vi "Auto Loop 4.vi"(2 "Auto State":u8, 3 "Call Context":T1) -> (1 "SubState 5":T2)   [LabVIEW 2014]
uses:
  typedefs/state machine/singleUseSubstate.ctl
  <vilib>/Rock Robotics/WPI/DriverStation/WPI_DriverStationDerivedRobotMode.ctl
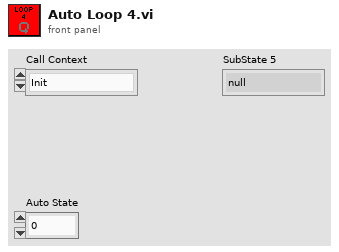
[diagram p1: front panel]
types:
  T1 = typedef "WPI_DriverStationDerivedRobotMode.ctl" = enum16{"Init", "Execute", "Stop"}
  T2 = typedef "singleUseSubstate.ctl" = enum16{"null", "wait", "shift high", "shift low", "end"}
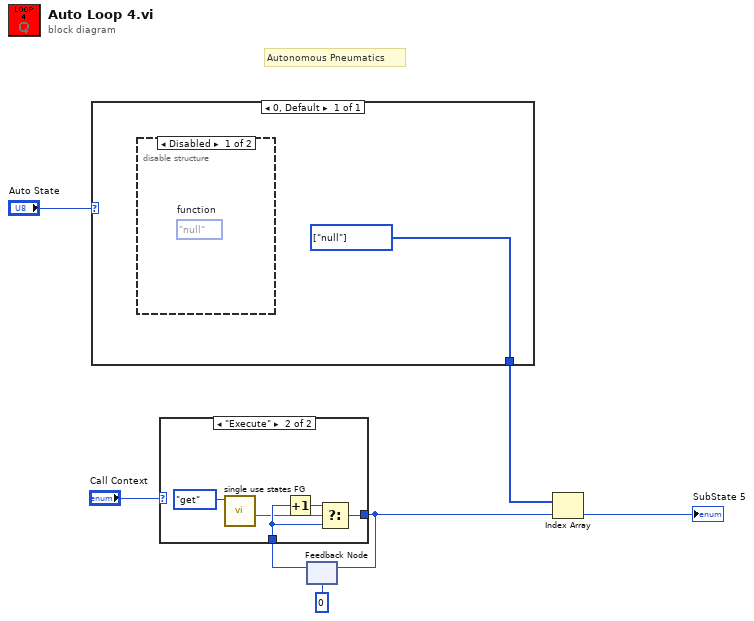
[diagram p0: block diagram]
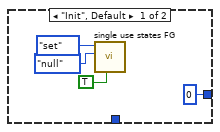
[diagram p3: hidden frame]
diagram:
  # "Autonomous Pneumatics"
  n1 = case shown="0, Default" "Auto State" {
    tunnel: [w8] -> w5
    frame 0, Default {
      w8 = T2[] [enum."null"] items=["null", "wait", "shift high", "shift low", "end"]
      n2 = disable-structure shown="Disabled" {
        frame Disabled {
          (unwired) singleUseSubstate."null"  # function
        }
        frame Enabled {
        }
      }
    }
  }
  n3 = feedback #1(0) -> (w7:i32)
  n4 = case shown="\"Execute\"" "Call Context" {
    tunnel: w7 -> [_ w17]
    tunnel: [0 w16] -> w6
    frame "Init", Default {
      n5 = call "single use states FG.vi"("exit in"=TRUE, "substate"=singleUseSubstate."null", "menu (get)"=enum16{"set", "get"}."set") -> ()  [unwired: 5 in, 4 out]
    }
    frame "Execute" {
      n6 = call "single use states FG.vi"("menu (get)"=enum16{"set", "get"}."get") -> ("exit out"=w15:bool)  [unwired: 7 in, 3 out]
      n7 = Increment(x=w17) -> (x+1=w13:i32)
      n8 = Select(t=w13, s=w15, f=w17) -> (s? t:f=w16:i32)
    }
  }
  n9 = feedback-in #1(w6) -> ()
  n10 = Index Array(array=w5, index=w6) -> (element=→"SubState 5":T2)
